vi "setRowMinimumHeight.vi"(8 "Error In":errorcluster, 9 "minSize":i32, 10 "row":i32, 11 "QGridLayout In":refnum<class "QGridLayout.lvclass">) -> (0 "Error Out":errorcluster, 3 "QGridLayout Out":refnum<class "QGridLayout.lvclass">)   [LabVIEW 2014, in "QGridLayout.lvclass"]
doc: "LabVIEW-specific documentation is not yet available. See <b>https://doc.qt.io/qt-5/qgridlayout.html#setRowMinimumHeight</b>"
uses:
  QGridLayout.lvclass
  LQ Core/LQIdentity/LQIdentity.lvclass/LQIdentity.ctl
  LQ Core/LQ Core.lvlib
  LQ Core/LQIdentity/LQIdentity.lvclass
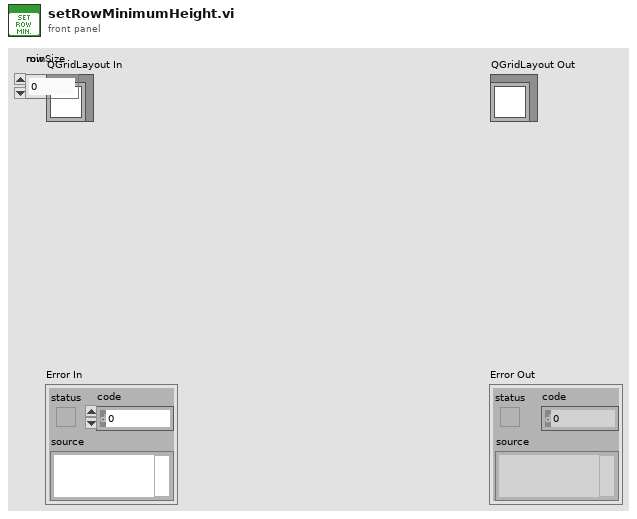
[diagram p1: front panel]
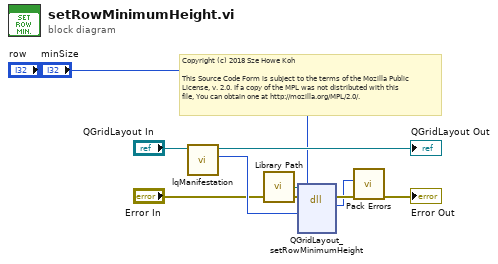
[diagram p0: block diagram]
diagram:
  # "Copyright (c) 2018 Sze Howe Koh\n\nThis Source Code Form is subject to the terms of the Mozilla Public\nLicense, v. 2.0. If a copy of the MPL was not distributed with this\nfile, You can obtain one at http://mozilla.org/MPL/2.0/."
  n1 = call "lqManifestation.vi"("LQIdentity in"="QGridLayout In") -> ("Manifestation"=w7:u64, "LQIdentity out"=→"QGridLayout Out":refnum<class "QGridLayout.lvclass">)  [unwired: 9 in]
  n2 = call "Library Path.vi"() -> ("Library Path"=w8:path)
  n3 = dll-call lib="?" fn="QGridLayout_setRowMinimumHeight"(path in=w8, error in="Error In", "_instance"=w7, "row"="row", "minSize"="minSize") -> (error out=w5:errorcluster, w3:i32)  [unwired: 4 in, 1 out]
  n4 = call "Pack Errors.vi"("Error In"=w5, "Error Code"=w3) -> ("Error Out"=→"Error Out":errorcluster)  [unwired: 9 in]
